vi "Instance to Map Entry.vi"(0 "MVA Comms VI in":refnum<class "MVA Comms VI Instance.lvclass">, 5 "Node Tests":refnum<class "Node Test.lvclass">[](array[class]), 11 "error in (no error)":errorcluster) -> (4 "MVA Comms VI out":refnum<class "MVA Comms VI Instance.lvclass">, 6 "Map Key":T2[](array[typedef]), 8 "Array":T1[](array[typedef]), 15 "error out":errorcluster)   [LabVIEW 2020, in "MVA Message Mapper.lvlib" / "MVA Comms VI Instance.lvclass"]
uses:
  <vilib>/gpm_packages/@cs/Bus-message-mapper/Source/support/MVA Comms/MVA Comms VI Instance.lvclass
  <vilib>/gpm_packages/@cs/Bus-message-mapper/Source/controls/Map Key.ctl
  <vilib>/gpm_packages/@cs/Bus-message-mapper/Source/controls/Datum Endpoint.ctl
  <vilib>/gpm_packages/@cs/Bus-message-mapper/Source/support/Traversal Algorithm/Node Test.lvclass
  <vilib>/gpm_packages/@cs/Bus-message-mapper/Source/support/MVA Comms/MVA Comms VI Instance.lvclass/MVA Comms VI Instance.ctl
  <vilib>/gpm_packages/@cs/Bus-message-mapper/Source/support/MVA Comms/Accessors/Read MVA Coms VI Instance.vi
  <vilib>/gpm_packages/@cs/Bus-message-mapper/Source/support/MVA Comms/Accessors/Read MVA Object In Terminal.vi
  <vilib>/gpm_packages/@cs/Bus-message-mapper/Source/support/MVA Comms/Accessors/Read Datum Value Terminal.vi
  <vilib>/gpm_packages/@cs/Bus-message-mapper/Source/support/MVA Comms/Accessors/Read Datum Name Terminal.vi
  <vilib>/gpm_packages/@cs/Bus-message-mapper/Source/support/MVA Comms/Accessors/Read MVA Coms VI Name.vi
  <vilib>/gpm_packages/@cs/Bus-message-mapper/Source/MVA Message Mapper.lvlib
  <vilib>/Utility/Data Type/NI_Data Type.lvlib
  <vilib>/gpm_packages/@cs/variant/Source/VariantExtensions.lvlib
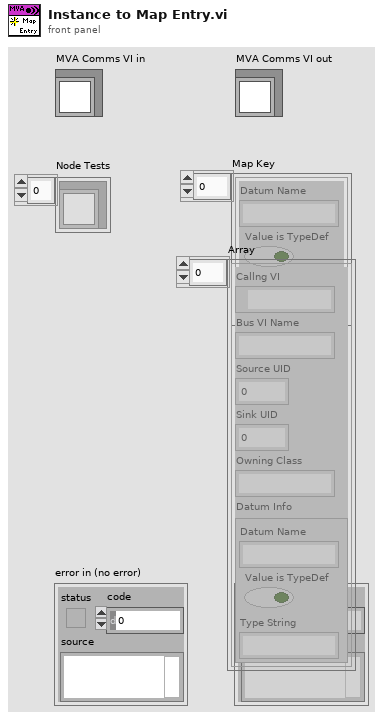
[diagram p1: front panel]
types:
  T1 = typedef "MVA Message Mapper.lvlib/Datum Endpoint.ctl" = cluster{"Callng VI":path, "Bus VI Name":string, "Source UID":i32, "Sink UID":i32, "Owning Class":string, "Datum Info":T2}
  T2 = typedef "MVA Message Mapper.lvlib/Map Key.ctl" = cluster{"Datum Name":string, "Value is TypeDef":bool, "Type String":string}
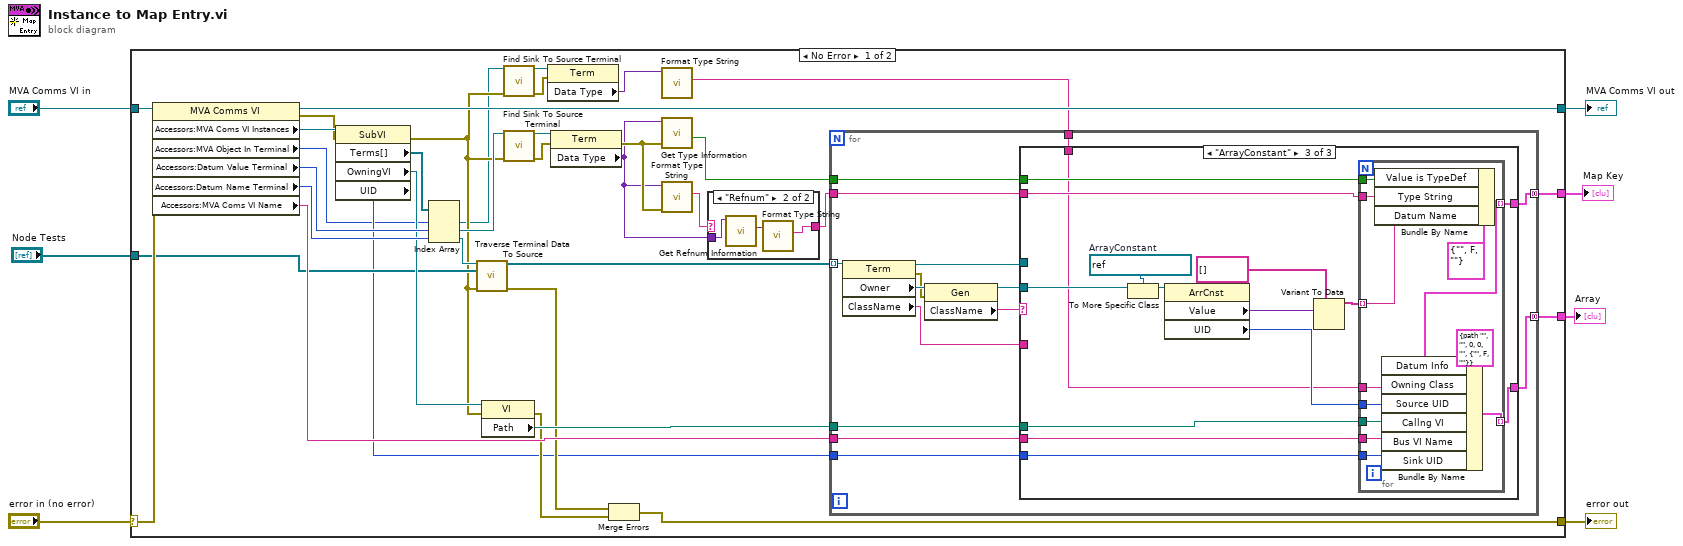
[diagram p0: block diagram]
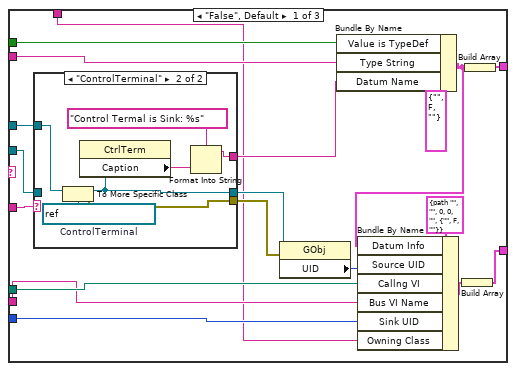
[diagram p3: hidden frame]
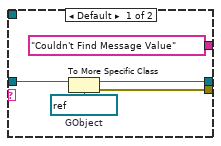
[diagram p4: hidden frame]
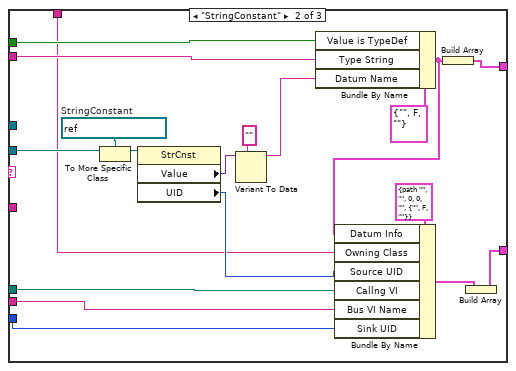
[diagram p5: hidden frame]
diagram:
  n1 = case shown="No Error" "error in (no error)" {
    selector: "error in (no error)" -> [w30 w140]
    tunnel: [w26 w140] -> w6
    tunnel: [w41 w139] -> w4
    tunnel: "MVA Comms VI in" -> [w42 w139]
    tunnel: [w35 _] -> w3
    tunnel: "Node Tests" -> [w21 _]
    tunnel: [w20 _] -> w1
    frame No Error {
      n2 = property class="MVA Comms VI"(reference=w42, error in=w30) -> (reference out=w41:refnum<class "MVA Comms VI Instance.lvclass">, error out=w29:errorcluster, "Accessors:MVA Coms VI Instances"=w38:refnum<vi>, "Accessors:MVA Object In Terminal"=w14:i32, "Accessors:Datum Value Terminal"=w37:i32, "Accessors:Datum Name Terminal"=w36:i32, "Accessors:MVA Coms VI Name"=w32:string)
      n3 = property class="SubVI"(reference=w38, error in=w29) -> (error out=w12:errorcluster, "Terms[]"=w40:refnum<vi>[], "OwningVI"=w33:refnum<vi>, "UID"=w16:i32)  [unwired: 1 out]
      n4 = Index Array(array=w40, index #1=w14, index #2=w37, index #3=w36) -> (element #1=w10:refnum<vi>, element #2=w25:refnum<vi>, element #3=w39:refnum<vi>)
      n5 = call <vilib>:"Traverse Terminal Data To Source.vi"("Terminal in"=w39, "Node Tests"=w21, "error in (no error)"=w12) -> ("Source Terminals"=w34:refnum<vi>[], "error out"=w27:errorcluster)  [unwired: 11 in]
      n6 = property class="VI"(reference=w33, error in=w12) -> (error out=w28:errorcluster, "Path"=w31:path)  [unwired: 1 out]
      n7 = call <vilib>:"Find Sink To Source Terminal.vi"("Source Terminal"=w10, "error in (no error)"=w12) -> ("Sink Terminal"=w13:refnum<vi>, "error out"=w11:errorcluster)  [unwired: 12 in]
      n8 = call <vilib>:"Find Sink To Source Terminal.vi"("Source Terminal"=w25, "error in (no error)"=w12) -> ("Sink Terminal"=w15:refnum<vi>, "error out"=w23:errorcluster)  [unwired: 12 in]
      n9 = property on="Property Node" class="Term"(reference=w13, error in=w11) -> ("Data Type"=w9:variant)  [unwired: 2 out]
      n10 = property on="Property Node" class="Term"(reference=w15, error in=w23) -> (error out=w22:errorcluster, "Data Type"=w18:variant)  [unwired: 1 out]
      n11 = Merge Errors(w27, w28) -> (w26:errorcluster)
      n12 = call <vilib>:"Format Type String.vi"("Data Type"=w9) -> ("Type Name"=w8:string)  [unwired: 9 in, 1 out]
      n13 = call <vilib>:"Get Type Information.vi"("error in (no error)"=w22, "variant"=w18) -> ("type definition"=w24:bool)  [unwired: 5 in, 4 out]
      n14 = call <vilib>:"Format Type String.vi"("error in (no error)"=w22, "Data Type"=w18) -> ("Type Name"=w19:string)  [unwired: 8 in, 1 out]
      n15 = case shown="\"Refnum\"" w19 {
        selector: w19 -> [w43 _]
        tunnel: w18 -> [_ w46]
        tunnel: [w43 w44] -> w17
        frame "False", Default {
        }
        frame "Refnum" {
          n16 = call <vilib>:"Get Refnum Information.vi"("variant"=w46) -> ("strict type"=w45:variant)  [unwired: 7 in, 3 out]
          n17 = call <vilib>:"Format Type String.vi"("Data Type"=w45) -> ("Type Name"=w44:string)  [unwired: 9 in, 1 out]
        }
      }
      n18 = for {
        tunnel: [w54] -> w35 mode=concatenating
        tunnel: w34 -> [w60] mode=indexing
        tunnel: w32 -> [w52]
        tunnel: w31 -> [w53]
        tunnel: w24 -> [w56]
        tunnel: w17 -> [w55]
        tunnel: [w51] -> w20 mode=concatenating
        tunnel: w16 -> [w50]
        tunnel: w8 -> [w47]
        n19 = property on="Property Node" class="Term"(reference=w60) -> (reference out=w48:refnum<vi>, error out=w58:errorcluster, "Owner"=w61:refnum<vi>, "ClassName"=w49:string)  [unwired: 1 in]
        n20 = property on="Property Node" class="Gen"(reference=w61, error in=w58) -> (reference out=w57:refnum<vi>, "ClassName"=w59:string)  [unwired: 1 out]
        n21 = case shown="\"ArrayConstant\"" w59 {
          tunnel: w57 -> [w79 w107 w123]
          tunnel: w56 -> [w76 w104 w121]
          tunnel: w55 -> [w77 w105 w120]
          tunnel: [w75 w102 w118] -> w54
          tunnel: w53 -> [w72 w99 w117]
          tunnel: w52 -> [w71 w98 w116]
          tunnel: [w69 w96 w114] -> w51
          tunnel: w50 -> [w68 w95 w113]
          tunnel: w49 -> [w66 _ _]
          tunnel: w48 -> [w65 _ _]
          tunnel: w47 -> [w63 w94 w112]
          frame "False", Default {
            n22 = case shown="\"ControlTerminal\"" w66 {
              tunnel: [w85 w87] -> w80
              tunnel: w79 -> [w83 _]
              tunnel: [w82 w90] -> w67
              tunnel: w65 -> [_ w91]
              tunnel: ["Couldn't Find Message Value" w88] -> w64
              frame Default {
                w84 = refnum<vi> refnum  # GObject
                n23 = To More Specific Class(target class=w84, reference=w83) -> (specific class reference=w85:refnum<vi>, error out=w82:errorcluster)  [unwired: 1 in]
              }
              frame "ControlTerminal" {
                w92 = refnum<vi> refnum  # ControlTerminal
                n24 = To More Specific Class(target class=w92, reference=w91) -> (specific class reference=w87:refnum<vi>, error out=w90:errorcluster)  [unwired: 1 in]
                n25 = property on="Property Node" class="CtrlTerm"(reference=w87) -> ("Caption"=w86:string)  [unwired: 1 in, 2 out]
                n26 = Format Into String(format string="Control Termal is Sink: %s", w86) -> (resulting string=w88:string)  [unwired: 2 in, 1 out]
              }
            }
            n27 = property class="GObj"(reference=w80, error in=w67) -> ("UID"=w73:i32)  [unwired: 2 out]
            n28 = Bundle By Name(cluster=T2 {"Datum Name"="", "Value is TypeDef"=FALSE, "Type String"=""} ("Map Key"), "Value is TypeDef"=w76, "Type String"=w77, "Datum Name"=w64) -> (w62:T2)
            n29 = Bundle By Name(cluster=T1 {"Callng VI"=path "", "Bus VI Name"="", "Source UID"=0, "Sink UID"=0, "Owning Class"="", "Datum Info"={"Datum Name"="", "Value is TypeDef"=FALSE, "Type String"=""}} ("Set Value"), "Datum Info"=w62, "Source UID"=w73, "Callng VI"=w72, "Bus VI Name"=w71, "Sink UID"=w68, "Owning Class"=w63) -> (w70:T1)
            n30 = Build Array(w70) -> (w69:T1[])
            n31 = Build Array(w62) -> (w75:T2[])
          }
          frame "StringConstant" {
            w111 = refnum<vi> refnum  # StringConstant
            n32 = To More Specific Class(target class=w111, reference=w107) -> (specific class reference=w110:refnum<vi>)  [unwired: 1 in, 1 out]
            n33 = property class="StrCnst"(reference=w110) -> ("Value"=w109:variant, "UID"=w100:i32)  [unwired: 1 in, 2 out]
            n34 = Variant To Data(type="", Variant=w109) -> (data=w106:string)  [unwired: 1 in, 1 out]
            n35 = Bundle By Name(cluster=T2 {"Datum Name"="", "Value is TypeDef"=FALSE, "Type String"=""} ("Map Key"), "Value is TypeDef"=w104, "Type String"=w105, "Datum Name"=w106) -> (w93:T2)
            n36 = Bundle By Name(cluster=T1 {"Callng VI"=path "", "Bus VI Name"="", "Source UID"=0, "Sink UID"=0, "Owning Class"="", "Datum Info"={"Datum Name"="", "Value is TypeDef"=FALSE, "Type String"=""}} ("Set Value"), "Datum Info"=w93, "Owning Class"=w94, "Source UID"=w100, "Callng VI"=w99, "Bus VI Name"=w98, "Sink UID"=w95) -> (w97:T1)
            n37 = Build Array(w93) -> (w102:T2[])
            n38 = Build Array(w97) -> (w96:T1[])
          }
          frame "ArrayConstant" {
            w126 = refnum<vi> refnum  # ArrayConstant
            n39 = To More Specific Class(target class=w126, reference=w123) -> (specific class reference=w125:refnum<vi>)  [unwired: 1 in, 1 out]
            n40 = property class="ArrCnst"(reference=w125) -> ("Value"=w124:variant, "UID"=w115:i32)  [unwired: 1 in, 2 out]
            n41 = Variant To Data(type=string[] [], Variant=w124) -> (data=w119:string[])  [unwired: 1 in, 1 out]
            n42 = for {
              tunnel: w121 -> [w137]
              tunnel: w120 -> [w136]
              tunnel: w119 -> [w135] mode=indexing
              tunnel: [w127] -> w118 mode=indexing
              tunnel: w117 -> [w133]
              tunnel: w116 -> [w132]
              tunnel: w115 -> [w131]
              tunnel: [w130] -> w114 mode=indexing
              tunnel: w113 -> [w129]
              tunnel: w112 -> [w128]
              n43 = Bundle By Name(cluster=T2 {"Datum Name"="", "Value is TypeDef"=FALSE, "Type String"=""} ("Map Key"), "Value is TypeDef"=w137, "Type String"=w136, "Datum Name"=w135) -> (w127:T2)
              n44 = Bundle By Name(cluster=T1 {"Callng VI"=path "", "Bus VI Name"="", "Source UID"=0, "Sink UID"=0, "Owning Class"="", "Datum Info"={"Datum Name"="", "Value is TypeDef"=FALSE, "Type String"=""}} ("Set Value"), "Datum Info"=w127, "Owning Class"=w128, "Source UID"=w131, "Callng VI"=w133, "Bus VI Name"=w132, "Sink UID"=w129) -> (w130:T1)
            }
          }
        }
      }
    }
    frame Error {
    }
  }
  "error out" <- w6
  "MVA Comms VI out" <- w4
  "Map Key" <- w3
  "Array" <- w1
